vi "AD7609 Check overrun.vi"() -> (1 "Overruns":u32, 2 "Overrun error out":errorcluster)   [LabVIEW 2014]
uses:
  <vilib>/Instr/_visa.llb/VISA Open Access Mode.ctl
  <vilib>/Instr/_visa.llb/VISA Configure Serial Port (Instr).vi
  AD7609 global.vi
panel:
  out "Overrun string output":string
  # "PN 25/11/2014"
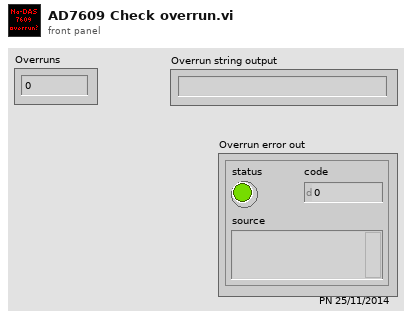
[diagram p1: front panel]
types:
  T1 = typedef "VISA Open Access Mode.ctl" = u32
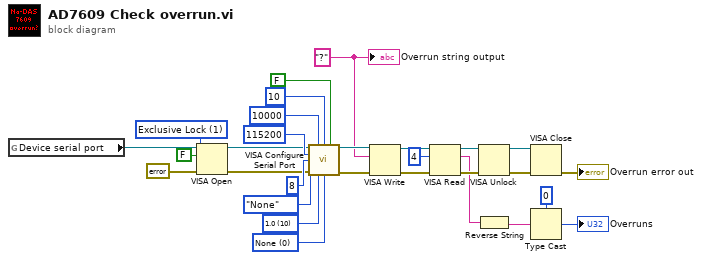
[diagram p0: block diagram]
diagram:
  w21 = T1 1 items=["VISA Defaults"=0, "Exclusive Lock"=1, "Load Configured Settings"=4] ("Access Mode")
  w22 = u16 0 items=["None", "XON/XOFF", "RTS/CTS", "XON/XOFF & RTS/CTS", "DTR/DSR", "XON/XOFF & DTR/DSR"] ("flow control (0:none)")
  w23 = u16 10 items=["1.0"=10, "1.5"=15, "2.0"=20] ("stop bits (10: 1 bit)")
  w10 = "?"
  n1 = global read "AD7609 global.vi" "Device serial port"() -> (w11:refnum<visa-resource-name>)
  n2 = VISA Open(duplicate session (F)=FALSE, access mode=w21, error in (no error)=errorcluster {"status"=FALSE, "code"=0, "source"=""}, VISA resource name=w11) -> (VISA resource name=w14:refnum<visa-resource-name>, error out=w16:errorcluster)  [unwired: 1 in]
  n3 = call-poly "VISA Configure Serial Port"("VISA resource name"=w14, "timeout (10sec)"=u32 10000, "termination char\n(0xA = '\\n' = LF)"=u8 10 ("termination char\n(0xA = '\\n' = LF)"), "Enable Termination\nChar (T)"=FALSE ("Enable Termination\nChar (T)"), "baud rate (9600)"=u32 115200, "data bits (8)"=u16 8, "parity (0:none)"=enum16{"None", "Odd", "Even", "Mark", "Space"}."None", "error in (no error)"=w16, "stop bits (10: 1 bit)"=w23, "flow control (0:none)"=w22) -> ("VISA resource name out"=w13:refnum<visa-resource-name>, "error out"=w15:errorcluster)  [unwired: 4 in]
  n4 = VISA Write(VISA resource name=w13, write buffer=w10, error in (no error)=w15) -> (VISA resource name out=w6:refnum<visa-resource-name>, error out=w9:errorcluster)  [unwired: 1 out]
  n5 = VISA Read(VISA resource name=w6, byte count=u32 4, error in (no error)=w9) -> (VISA resource name out=w5:refnum<visa-resource-name>, read buffer=w3:string, error out=w8:errorcluster)  [unwired: 1 out]
  n6 = VISA Unlock(8:w8, 11:w5) -> (0:w18:errorcluster, 3:w19:refnum<visa-resource-name>)
  n7 = Reverse String(1:w3) -> (0:w1:string)
  n8 = VISA Close(VISA resource name=w19, error in (no error)=w18) -> (error out=→"Overrun error out":errorcluster)
  n9 = Type Cast(type=u32 0, x=w1) -> (*(type *) &x=→"Overruns":u32)
  "Overrun string output" <- w10
